vi "Wait on Execution.vi"(0 "Session Handle in":T1, 9 "Timeout mS (Forever)":i32=-1, 11 "error in (no error)":errorcluster) -> (4 "Session Handle out":T1, 8 "Timeout?":bool, 15 "error out":errorcluster)   [LabVIEW 2020, in "TSS.lvlib" / "Execution.lvclass"]
uses:
  Execution.lvclass
  Typedefs/Session Handle.ctl
  Get Execution Ref.vi
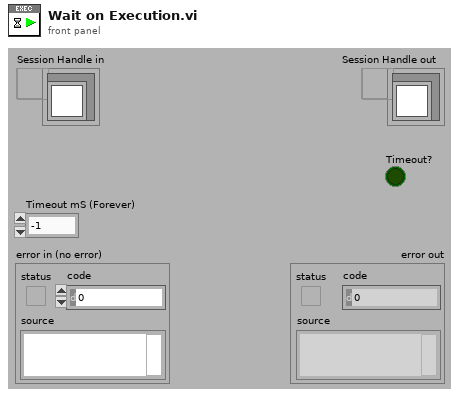
[diagram p1: front panel]
types:
  T1 = typedef "TSS.lvlib/Execution.lvclass/Session Handle.ctl" = refnum<data-value>
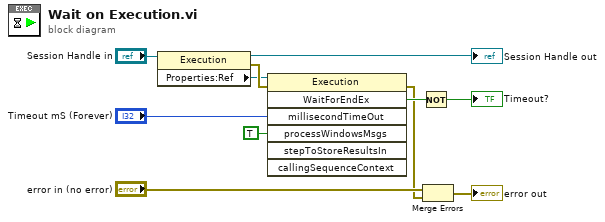
[diagram p0: block diagram]
diagram:
  n1 = property class="Execution"(reference="Session Handle in") -> (reference out=→"Session Handle out":T1, error out=w11:errorcluster, "Properties:Ref"=w8:refnum<k7>)  [unwired: 1 in]
  n2 = invoke class="Execution" method="WaitForEndEx"(reference=w8, error in=w11, "millisecondTimeOut"="Timeout mS (Forever)", "processWindowsMsgs"=TRUE) -> (error out=w2:errorcluster, "WaitForEndEx"=w5:bool)  [unwired: 3 in, 5 out]
  n3 = Not(x=w5) -> (.not. x?=→"Timeout?":bool)
  n4 = Merge Errors("error in (no error)", w2) -> (→"error out":errorcluster)
